vi "ADCP_Read_and_Update_Packets_From_Serial_Port_Emulator.vi"(8 "error in (no error)":errorcluster, 11 "ADCP In":refnum<class "ADCP.lvclass">) -> (0 "error out":errorcluster, 1 "Received Packet":u8[](array[numeric]), 2 "Packet Info":T1, 3 "ADCP out":refnum<class "ADCP.lvclass">)   [LabVIEW 2017, in "ADCP.lvclass"]
uses:
  ADCP.lvclass
  ADCP_Packet_Info.ctl
  ADCP.lvclass/ADCP.ctl
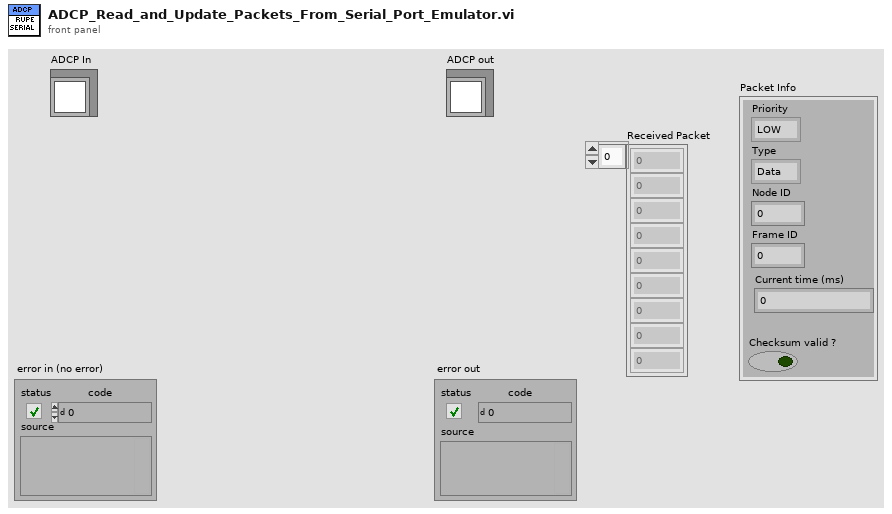
[diagram p1: front panel]
types:
  T1 = typedef "ADCP.lvclass/ADCP_Packet_Info.ctl" = cluster{"Priority":enum16{"LOW", "HIGH"}, "Type":enum16{"Data", "Connection Management", "Remote Request", "Error and status", "INVALID"}, "Node ID":i32, "Frame ID":i32, "Checksum valid ?":bool, "Current time (ms)":u32}
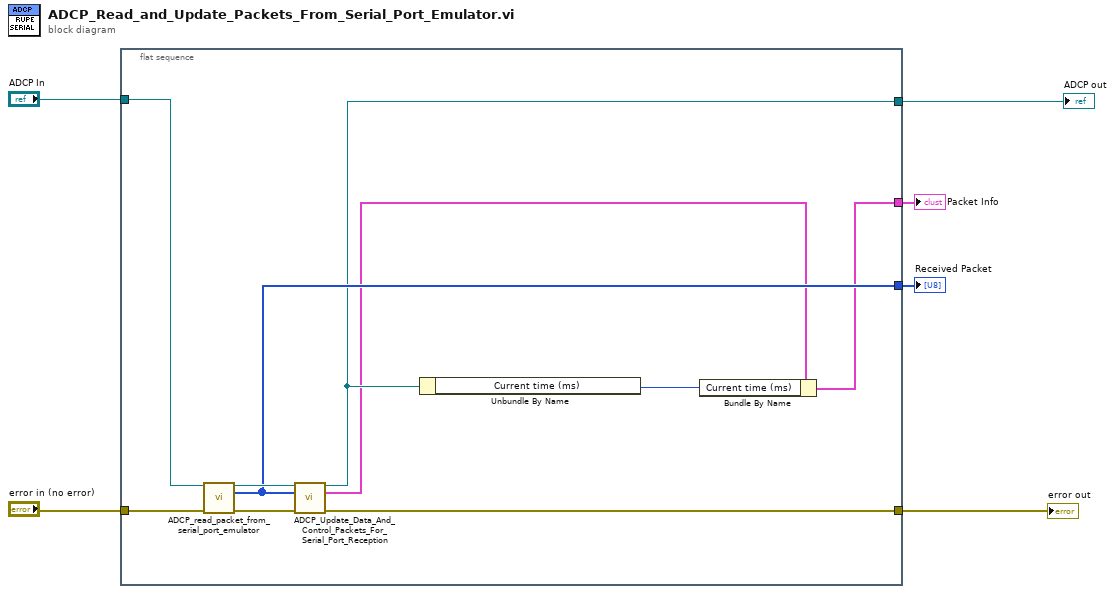
[diagram p0: block diagram]
diagram:
  n1 = flat-sequence {
    tunnel: "error in (no error)" -> [w16]
    tunnel: "ADCP In" -> [w15]
    tunnel: [w10] -> w4
    tunnel: [w12] -> w3
    tunnel: [w7] -> w2
    tunnel: [w11] -> w1
    frame #0 {
      n2 = call "ADCP_read_packet_from_serial_port_emulator.vi"("ADCP In"=w15, "error in (no error)"=w16) -> ("ADCP out"=w14:refnum<class "ADCP.lvclass">, "Received Packet"=w11:u8[], "error out"=w13:errorcluster)  [unwired: 6 in, 5 out]
      n3 = call "ADCP_Update_Data_And_Control_Packets_For_Serial_Port_Reception.vi"("ADCP In"=w14, "Processed Packet"=w11, "error in (no error)"=w13) -> ("ADCP out"=w10:refnum<class "ADCP.lvclass">, "Packet Info"=w8:T1, "error out"=w12:errorcluster)  [unwired: 10 in]
      n4 = Unbundle By Name(w10) -> ("Current time (ms)"=w9:u32)
      n5 = Bundle By Name(cluster=w8, "Current time (ms)"=w9) -> (w7:T1)
    }
  }
  "ADCP out" <- w4
  "error out" <- w3
  "Packet Info" <- w2
  "Received Packet" <- w1
